vi "Pattern recognizer.vi"() -> ()   [LabVIEW 2020]
uses:
  <vilib>/Native 3D Graph/xcontrol/3DPC_SurfacePlot.xctl
  controls/Pattern recognizer data.ctl
  cc2a312d-b526-45fa-be19-77dd4eded1a7.vi
  <vilib>/measure/mamon.llb/Waveform Peak Detection for 1 Chan.vi
  <vilib>/measure/NI_MAPro.lvlib
panel:
  in  "Tab Control":enum32{"Load", "Analyse"}(tab)
  in  "Messages":string
  in  "Fast load":bool=TRUE
  in  "Stop":bool
  out "Slicer view":cluster{"X":dbl, "Y":dbl}[](graph)
  in  "File Path":path
  in  "Load":bool
  out "3D Graph":refnum<class "Base Datatype.lvclass">[](xcontrol)
  in  "Width":i32=2
  in  "peaks/valleys":enum16{"Peaks", "Valleys"}(ring)
  in  "Threshold":dbl
  in  "Previous":bool
  in  "Next":bool
  in  "Loop count (0 for continuous)":u32
  in  "Generate":bool
  in  "Layer #":cluster{"Numeric":u32, "Numeric":u32}(slide)={"Numeric"=0, "Numeric"=480} scale=0.0..480.0
  out "Line# end":u32
  out "Line# start":u32
  out "End Gcode":string
  in  "Pattern":T1(ring)
  out "Pattern view":cluster{dbl[], dbl[]}[](graph)
  out "Start Gcode":string
  in  "Close":bool
  # "EXPERIMENTAL! Works like sh*t"
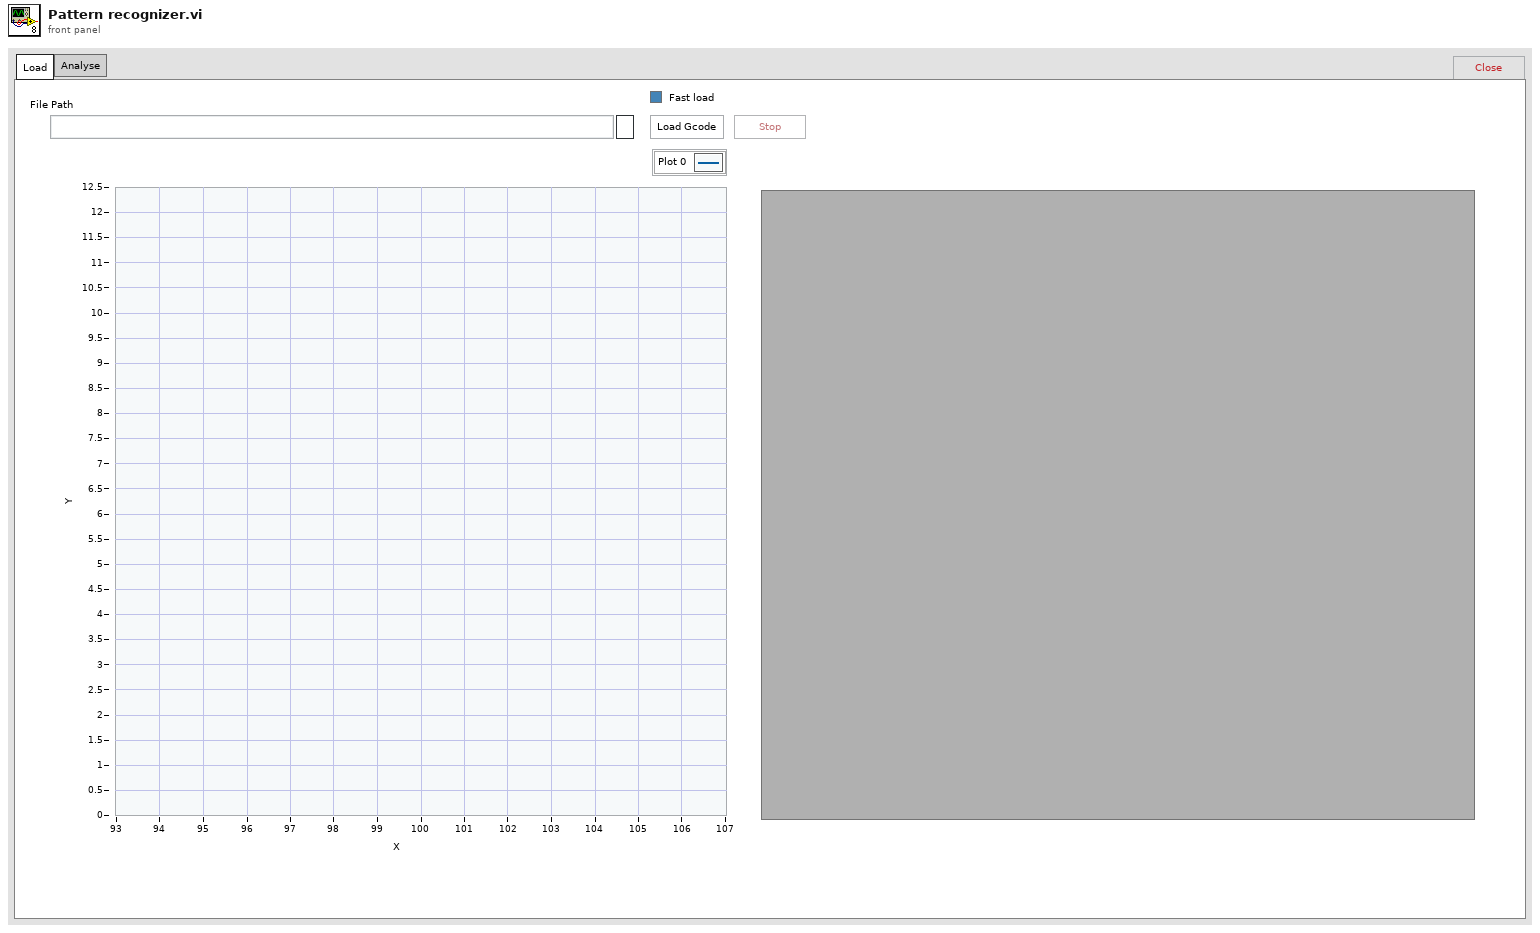
[diagram p1: front panel]
types:
  T1 = enum16{"X cumulative", "Y cumulative", "E cumulative", "X-Y absolute"}
  T2 = typedef "Pattern recognizer data.ctl" = cluster{"Gcode Array":string[], "Cumulative X":dbl[], "Cumulative Y":dbl[], "Cumulative E":dbl[], "Layer numbers":i32[], "Line number per layer":i32[]}
  T3 = enum8{"Enabled", "Disabled", "Disabled and Grayed Out"}
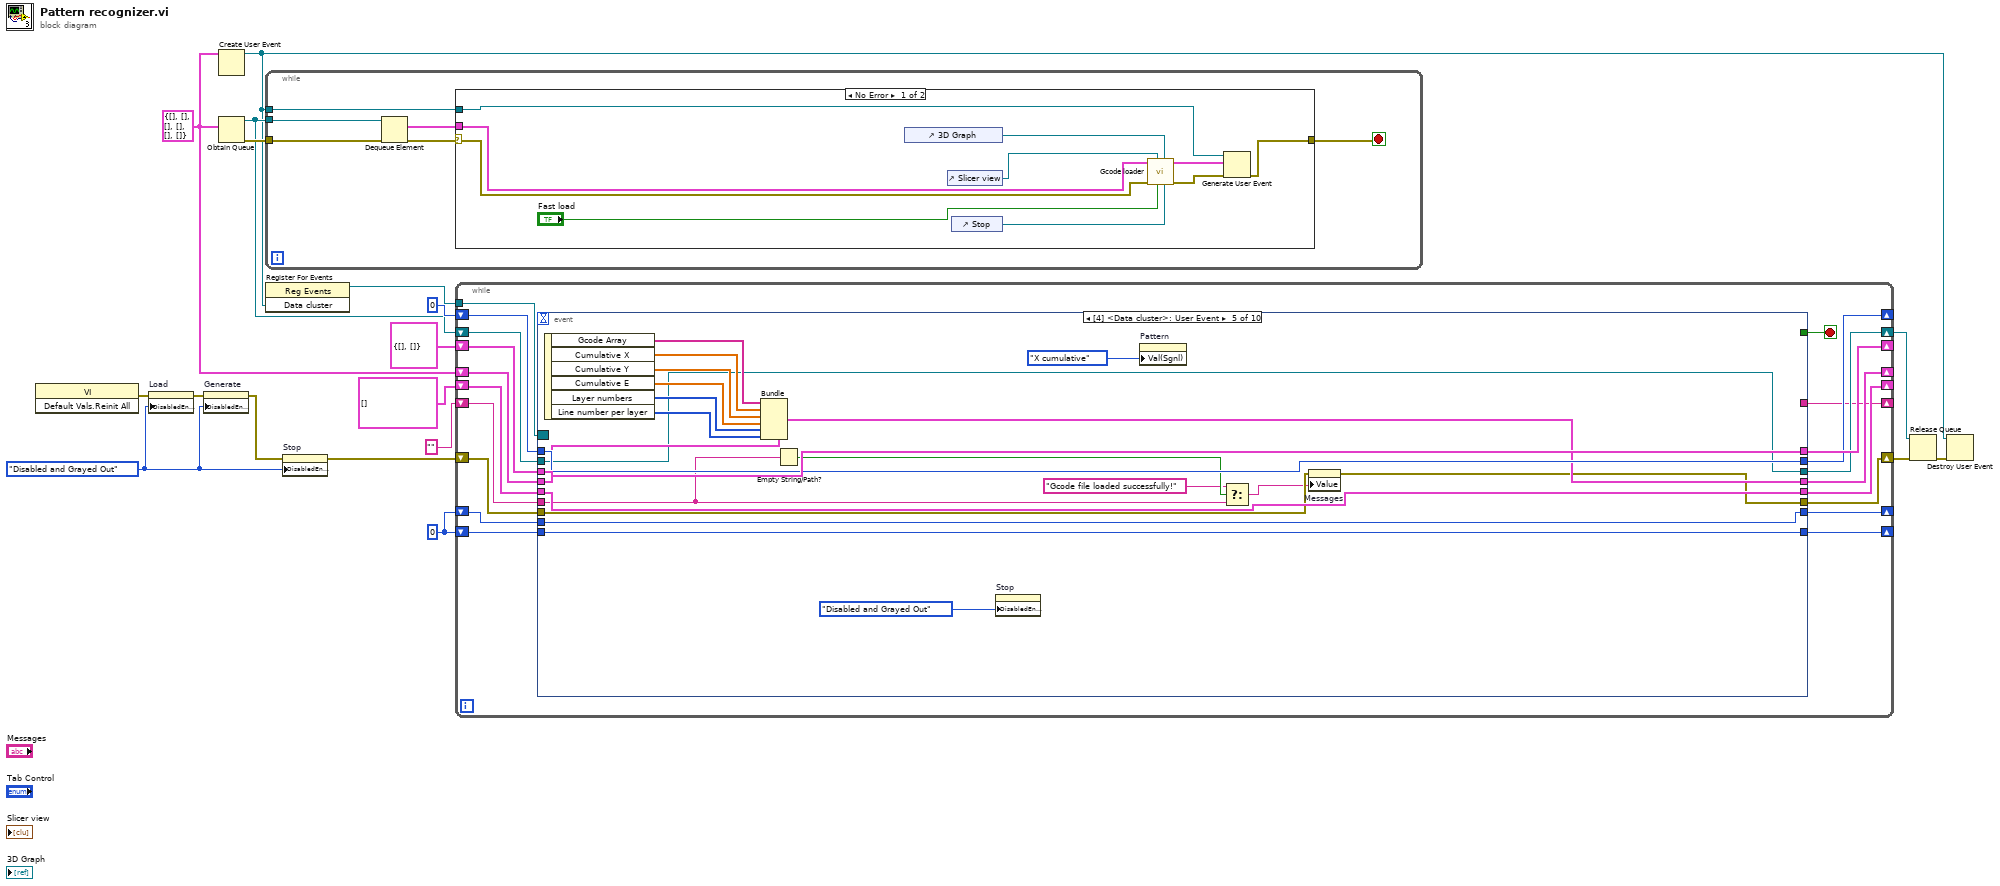
[diagram p0: block diagram]
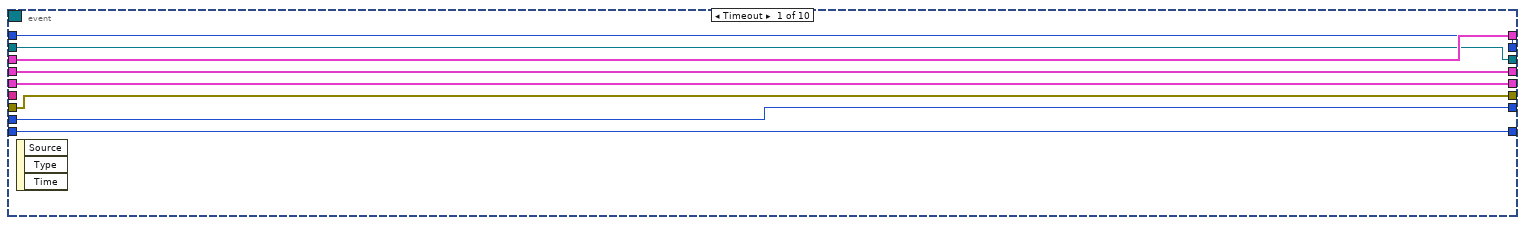
[diagram p3: hidden frame]
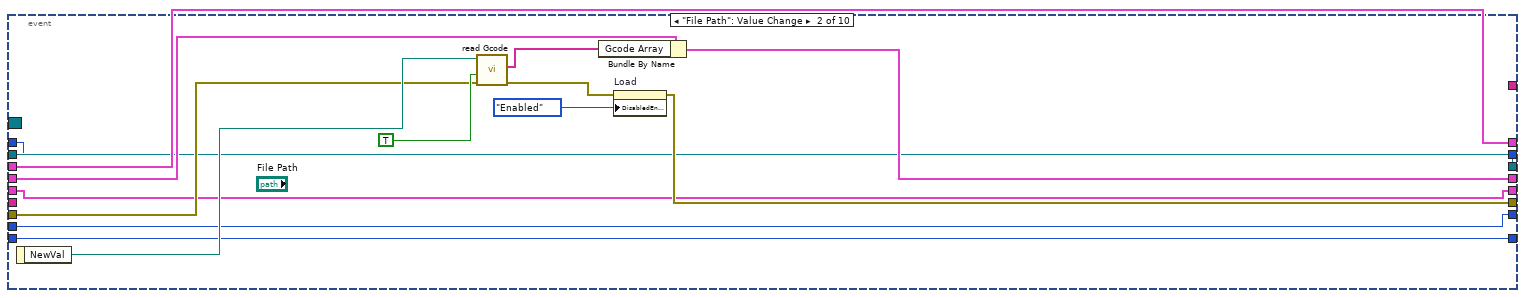
[diagram p4: hidden frame]
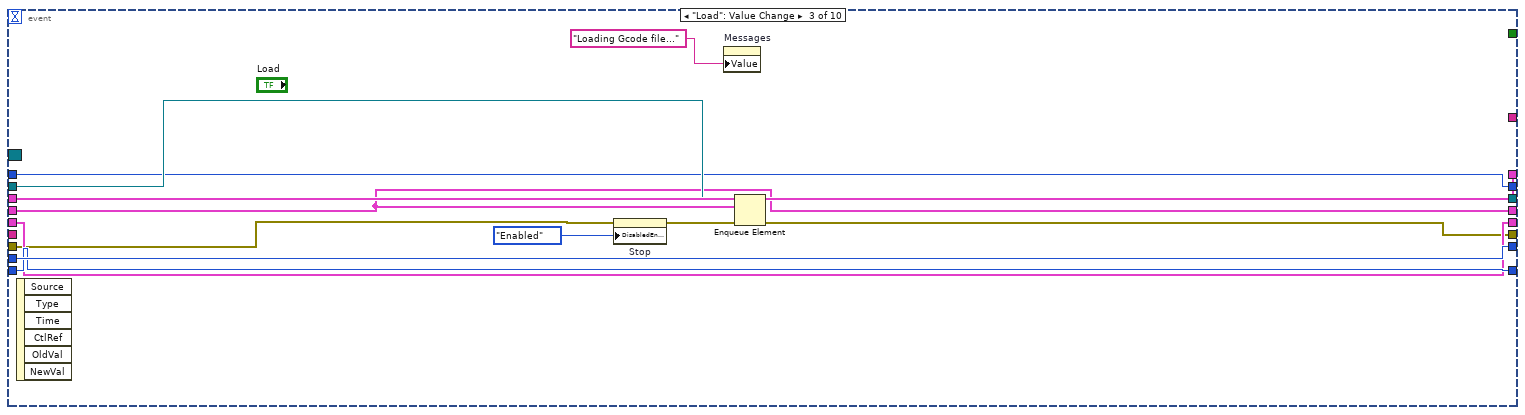
[diagram p5: hidden frame]
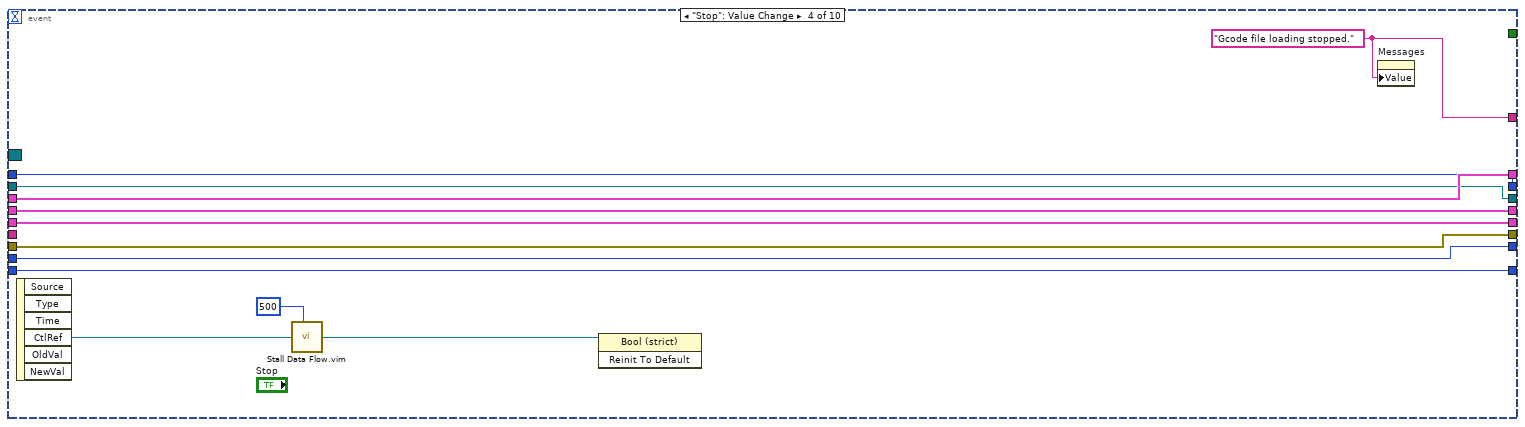
[diagram p6: hidden frame]
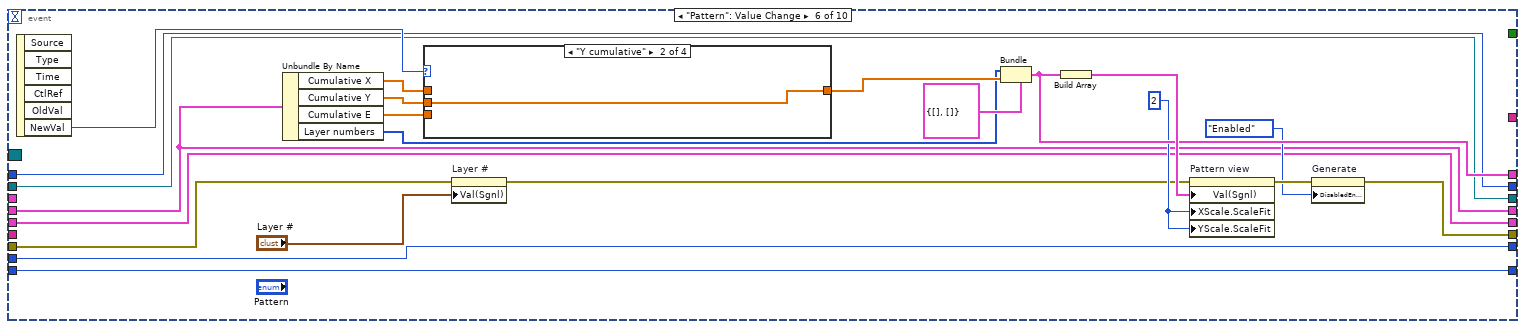
[diagram p7: hidden frame]
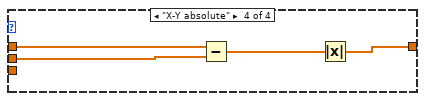
[diagram p10: hidden frame]
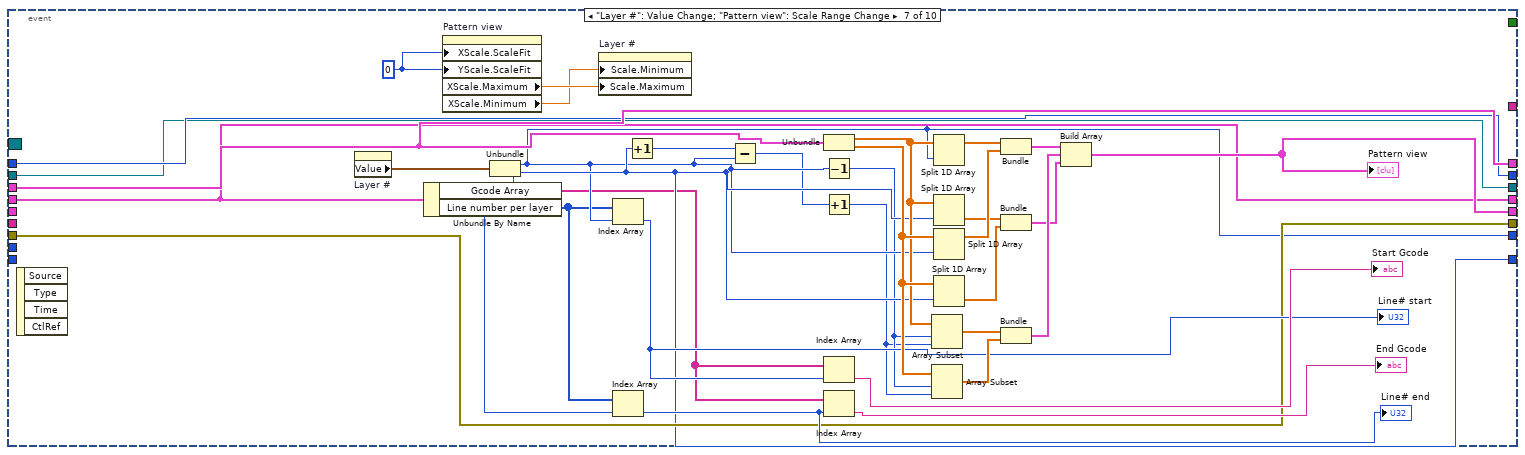
[diagram p11: hidden frame]
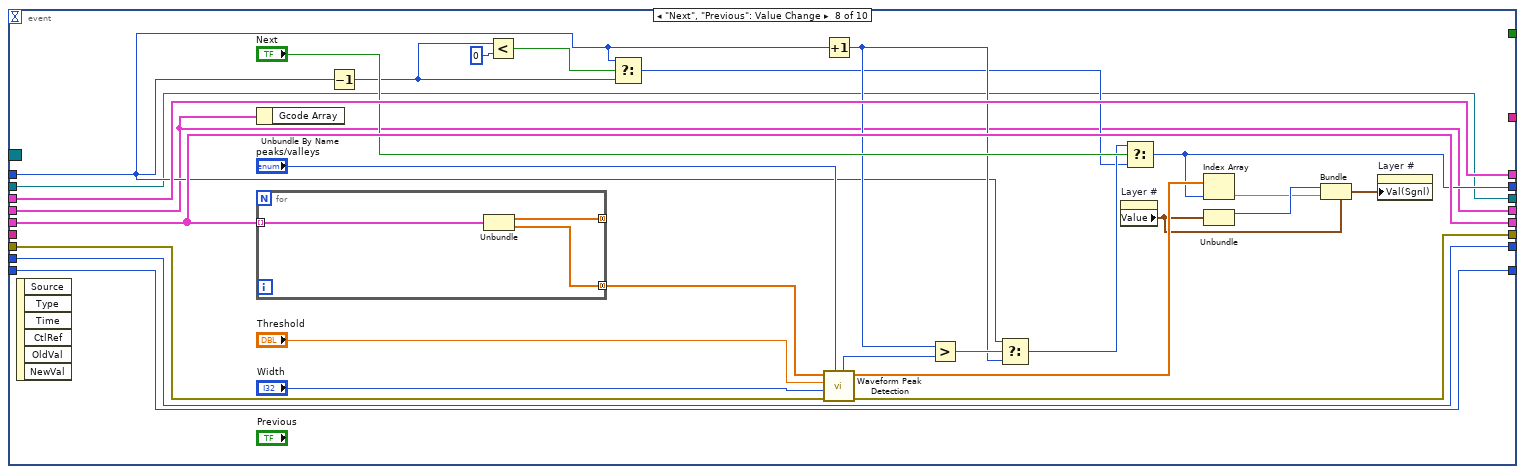
[diagram p12: hidden frame]
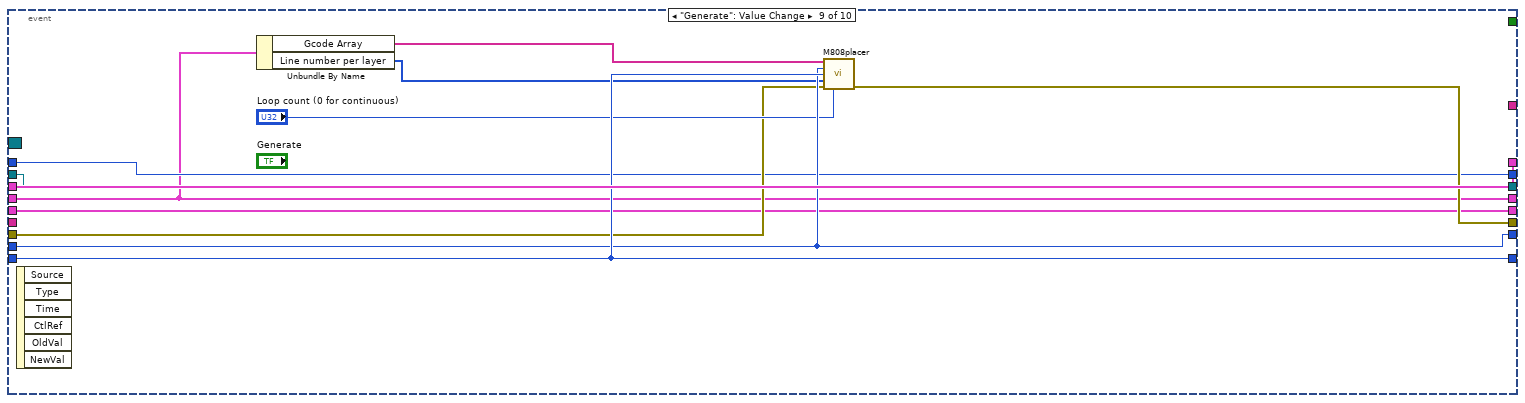
[diagram p13: hidden frame]
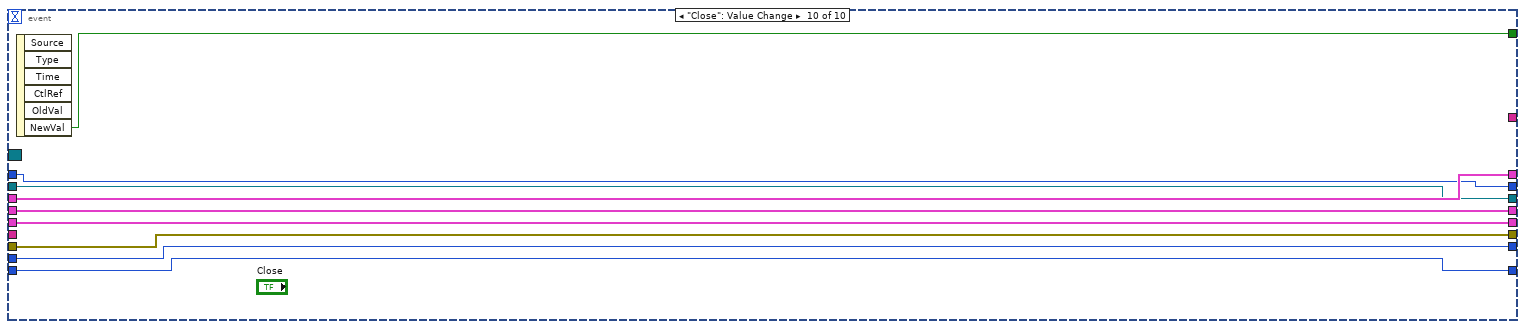
[diagram p14: hidden frame]
diagram:
  w11 = T2 {"Gcode Array"=[], "Cumulative X"=[], "Cumulative Y"=[], "Cumulative E"=[], "Layer numbers"=[], "Line number per layer"=[]} ("Data cluster")
  w3 = T3."Disabled and Grayed Out" ("Disabled")
  w17 = 0
  n1 = invoke class="VI" method="Default Vals.Reinit All"() -> (error out=w16:errorcluster)  [unwired: 3 in, 2 out]
  n2 = property on="Load" class="Bool"(error in=w16, "DisabledEnum"=w3) -> (error out=w15:errorcluster)  [unwired: 1 in, 1 out]
  n3 = property on="Generate" class="Bool"(error in=w15, "DisabledEnum"=w3) -> (error out=w2:errorcluster)  [unwired: 1 in, 1 out]
  n4 = Obtain Queue(element data type=w11) -> (queue out=w9:refnum<queue>, error out=w12:errorcluster)  [unwired: 4 in, 1 out]
  n5 = Create User Event(user event datatype=w11) -> (user event=w5:refnum<user-event>)  [unwired: 1 in, 1 out]
  n6 = while {
    tunnel: w9 -> [w24]
    tunnel: w12 -> [w23]
    tunnel: w5 -> [w19]
    stop <- w20 stop-if-true
    n7 = Dequeue Element(queue=w24, error in (no error)=w23) -> (element=w22:T2, error out=w21:errorcluster)  [unwired: 1 in, 2 out]
    n8 = case shown="No Error" w21 {
      selector: w21 -> [w33 w35]
      tunnel: w22 -> [w34 _]
      tunnel: [w27 w35] -> w20
      tunnel: w19 -> [w29 _]
      frame No Error {
        n9 = control-ref of="3D Graph"() -> (w32:refnum<vi>)
        n10 = control-ref of="Slicer view"() -> (w31:refnum<vi>)
        n11 = control-ref of="Stop"() -> (w26:refnum<vi>)
        n12 = call "Gcode loader.vi"("Stop"=w26, "3D Graph"=w32, "Fast load"="Fast load", "XYGraph in"=w31, "error in (no error)"=w33, "Data cluster"=w34) -> ("error out"=w30:errorcluster, "Data cluster out"=w28:T2)  [unwired: 4 in]
        n13 = Generate User Event(user event=w29, event data cluster=w28, error in=w30) -> (error out=w27:errorcluster)  [unwired: 1 in, 1 out]
      }
      frame Error {
      }
    }
  }
  n14 = register-events(w5) -> (reference out=w10:refnum<event-registration>)  [unwired: 2 in, 1 out]
  n15 = property on="Stop" class="Bool (strict)"(error in=w2, "DisabledEnum"=w3) -> (error out=w1:errorcluster)  [unwired: 1 in, 1 out]
  n16 = while {
    shift-right: [w54] -> _
    shift-left: cluster{dbl[], dbl[]} {[], []} -> [w53]
    shift-right: [w52] -> _
    shift-left: w17 -> [w50]
    shift-right: [w51] -> _
    shift-left: w17 -> [w49]
    shift-right: [w47] -> w7
    shift-left: w1 -> [w48]
    shift-right: [w46] -> _
    shift-left: cluster{dbl[], dbl[]}[] [] -> [w45]
    shift-right: [w43] -> _
    shift-left: 0 -> [w44]
    shift-right: [w41] -> _
    shift-left: w11 -> [w42]
    tunnel: w10 -> [w40]
    shift-right: [w38] -> w8
    shift-left: w9 -> [w39]
    shift-right: [w37] -> _
    shift-left: "" ("Messages") -> [w36]
    stop <- w55 stop-if-true
    n17 = event shown="[4] <Data cluster>: User Event" {
      selector: w40 -> [_ _ _ _ _ _ _ _ _ _]
      dyn-events: _ -> [_ _ _ _ _ _ _ _ _ _]
      timeout: _ -> [_ _ _ _ _ _ _ _ _ _]
      tunnel: [_ _ _ _ _ _ _ _ _ w239] -> w55
      tunnel: [w63 w77 w91 w103 w125 w143 w178 w215 w230 w238] -> w54
      tunnel: w53 -> [w63 w77 w91 w103 w125 _ w178 w215 w230 w238]
      tunnel: [w62 w75 w90 w102 w124 w139 w163 w214 w228 w237] -> w52
      tunnel: [w61 w74 w89 w101 w123 w138 w164 w213 w229 w236] -> w51
      tunnel: w50 -> [w62 w75 w90 w102 w124 w139 _ w214 w228 w237]
      tunnel: w49 -> [w61 w74 w89 w101 w123 w138 _ w213 w229 w236]
      tunnel: w48 -> [w60 w73 w80 w100 w110 w135 w167 w209 w226 w235]
      tunnel: [w60 w70 w85 w100 w109 w134 w167 w208 w225 w235] -> w47
      tunnel: [w59 w69 w88 w99 w122 w133 w166 w210 w224 w234] -> w46
      tunnel: w45 -> [w59 w69 w88 w99 w122 w133 _ w210 w224 w234]
      tunnel: w44 -> [w58 w64 w83 w98 w121 w132 w165 w202 w223 w233]
      tunnel: [w58 w64 w83 w98 w121 w132 w165 w192 w223 w233] -> w43
      tunnel: w42 -> [w57 w68 w86 w97 w120 w131 w157 w189 w222 w232]
      tunnel: [w57 w66 w86 w97 w113 w131 w157 w189 w222 w232] -> w41
      tunnel: w39 -> [w56 w65 w87 w96 w111 w126 w155 w188 w219 w231]
      tunnel: [w56 w65 w84 w96 w111 w126 w155 w188 w219 w231] -> w38
      tunnel: [_ _ _ w92 _ _ _ _ _ _] -> w37
      tunnel: w36 -> [_ _ _ _ w105 _ _ _ _ _]
      event Timeout {
        n18 = event-data() -> ()  [unwired: 1 in, 3 out]
      }
      event "File Path": Value Change {
        n19 = event-data() -> ("NewVal"=w78:path)  [unwired: 1 in]
        n20 = call "read Gcode.vi"("error in"=w73, "Parse comment lines"=TRUE, "Gcode path (use dialog)"=w78) -> ("error out"=w71:errorcluster, "Gcode Array"=w67:string[])  [unwired: 6 in, 1 out]
        n21 = Bundle By Name(cluster=w68, "Gcode Array"=w67) -> (w66:T2)
        n22 = property on="Load" class="Bool"(error in=w71, "DisabledEnum"=T3."Enabled" ("Disabled")) -> (error out=w70:errorcluster)  [unwired: 1 in, 1 out]
      }
      event "Load": Value Change {
        n23 = event-data() -> ()  [unwired: 1 in, 6 out]
        n24 = property on="Stop" class="Bool (strict)"(error in=w80, "DisabledEnum"=T3."Enabled" ("Disabled")) -> (error out=w79:errorcluster)  [unwired: 1 in, 1 out]
        n25 = property on="Messages" class="Str"("Value"="Loading Gcode file..." ("Messages")) -> ()  [unwired: 2 in, 2 out]
        n26 = Enqueue Element(queue=w87, element=w86, error in (no error)=w79) -> (queue out=w84:refnum<queue>, error out=w85:errorcluster)  [unwired: 1 in, 1 out]
      }
      event "Stop": Value Change {
        w92 = "Gcode file loading stopped." ("Messages")
        n27 = event-data() -> ("CtlRef"=w95:refnum<vi>)  [unwired: 1 in, 5 out]
        n28 = call "Stall Data Flow.vim"("value in"=w95, "milliseconds to wait"=u32 500) -> ("value out"=w94:refnum<vi>)  [unwired: 1 out]
        n29 = invoke class="Bool (strict)" method="Reinit To Default"(reference=w94) -> ()  [unwired: 2 in, 3 out]
        n30 = property on="Messages" class="Str"("Value"=w92) -> ()  [unwired: 2 in, 2 out]
      }
      event User Event {
        n31 = event-data() -> ("Gcode Array"=w119:string[], "Cumulative X"=w118:dbl[], "Cumulative Y"=w117:dbl[], "Cumulative E"=w116:dbl[], "Layer numbers"=w115:i32[], "Line number per layer"=w114:i32[])  [unwired: 1 in]
        n32 = Bundle(cluster=w120, "Gcode Array"=w119, "Cumulative X"=w118, "Cumulative Y"=w117, "Cumulative E"=w116, "Layer numbers"=w115, "Line number per layer"=w114) -> (w113:T2)
        n33 = Empty String/Path?(string/path=w105) -> (empty?=w108:bool)
        n34 = property on="Stop" class="Bool (strict)"("DisabledEnum"=T3."Disabled and Grayed Out" ("Disabled")) -> ()  [unwired: 2 in, 2 out]
        n35 = property on="Pattern" class="Enum (strict)"("Val(Sgnl)"=T1."X cumulative" ("Value (Signaling)")) -> ()  [unwired: 2 in, 2 out]
        n36 = Select(t="Gcode file loaded successfully!" ("Messages"), s=w108, f=w105) -> (s? t:f=w106:string)
        n37 = property on="Messages" class="Str"(error in=w110, "Value"=w106) -> (error out=w109:errorcluster)  [unwired: 1 in, 1 out]
      }
      event "Pattern": Value Change {
        w142 = u8 2 ("X Scale.Scale Fit")
        n38 = event-data() -> ("NewVal"=w147:T1)  [unwired: 1 in, 5 out]
        n39 = Unbundle By Name(w131) -> ("Cumulative X"=w130:dbl[], "Cumulative Y"=w129:dbl[], "Cumulative E"=w128:dbl[], "Layer numbers"=w127:i32[])
        n40 = case shown="\"Y cumulative\"" w147 {
          tunnel: [w148 w149 w150 w151] -> w145
          tunnel: w130 -> [w148 _ _ w154]
          tunnel: w129 -> [_ w149 _ w153]
          tunnel: w128 -> [_ _ w150 _]
          frame "X cumulative", Default {
          }
          frame "Y cumulative" {
          }
          frame "E cumulative" {
          }
          frame "X-Y absolute" {
            n41 = Subtract(x=w154, y=w153) -> (x-y=w152:dbl[])
            n42 = Absolute Value(x=w152) -> (abs(x)=w151:dbl[])
          }
        }
        n43 = property on="Layer #" class="Slide (strict)"(error in=w135, "Val(Sgnl)"="Layer #") -> (error out=w140:errorcluster)  [unwired: 1 in, 1 out]
        n44 = Bundle(cluster=cluster{dbl[], dbl[]} {[], []}, w127, w145) -> (w143:cluster{dbl[], dbl[]})
        n45 = Build Array(w143) -> (w144:cluster{dbl[], dbl[]}[])
        n46 = property on="Pattern view" class="XYGraph (strict)"(error in=w140, "Val(Sgnl)"=w144, "XScale.ScaleFit"=w142, "YScale.ScaleFit"=w142) -> (error out=w137:errorcluster)  [unwired: 1 in, 1 out]
        n47 = property on="Generate" class="Bool"(error in=w137, "DisabledEnum"=T3."Enabled" ("Disabled")) -> (error out=w134:errorcluster)  [unwired: 1 in, 1 out]
      }
      event "Layer #": Value Change; "Pattern view": Scale Range Change {
        w175 = u8 0 ("X Scale.Scale Fit")
        n48 = event-data() -> ()  [unwired: 1 in, 4 out]
        n49 = property on="Layer #" class="Slide (strict)"() -> ("Value"=w172:cluster{"Numeric":u32, "Numeric":u32})  [unwired: 2 in, 2 out]
        n50 = Unbundle By Name(w157) -> ("Gcode Array"=w158:string[], "Line number per layer"=w156:i32[])
        n51 = property on="Pattern view" class="XYGraph (strict)"("XScale.ScaleFit"=w175, "YScale.ScaleFit"=w175) -> ("XScale.Maximum"=w174:dbl, "XScale.Minimum"=w173:dbl)  [unwired: 2 in, 2 out]
        n52 = Unbundle(w172) -> ("Numeric"=w163:u32, "Numeric"=w164:u32)
        n53 = property on="Layer #" class="Slide (strict)"("Scale.Minimum"=w173, "Scale.Maximum"=w174) -> ()  [unwired: 2 in, 2 out]
        n54 = Index Array(array=w156, index=w163) -> (element=w169:i32)
        "Line# start" <- w169
        n55 = Index Array(array=w156, index=w164) -> (element=w168:i32)
        "Line# end" <- w168
        n56 = Increment(x=w164) -> (x+1=w161:u32)
        n57 = Subtract(x=w161, y=w163) -> (x-y=w162:u32)
        n58 = Unbundle(w178) -> (w176:dbl[], w177:dbl[])
        n59 = Decrement(x=w163) -> (x-1=w160:u32)
        n60 = Increment(x=w162) -> (x+1=w159:u32)
        n61 = Index Array(array=w158, index=w169) -> (element=→"Start Gcode":string)
        n62 = Index Array(array=w158, index=w168) -> (element=→"End Gcode":string)
        n63 = Array Subset(array=w176, index=w160, length=w159) -> (w180:dbl[])
        n64 = Array Subset(array=w177, index=w160, length=w159) -> (w179:dbl[])
        n65 = Split 1D Array(array=w176, index=w163) -> (first subarray=w187:dbl[])  [unwired: 1 out]
        n66 = Split 1D Array(array=w176, index=w164) -> (second subarray=w185:dbl[])  [unwired: 1 out]
        n67 = Split 1D Array(array=w177, index=w163) -> (first subarray=w186:dbl[])  [unwired: 1 out]
        n68 = Split 1D Array(array=w177, index=w164) -> (second subarray=w184:dbl[])  [unwired: 1 out]
        n69 = Bundle(w187, w186) -> (w183:cluster{dbl[], dbl[]})  [unwired: 1 in]
        n70 = Bundle(w185, w184) -> (w181:cluster{dbl[], dbl[]})  [unwired: 1 in]
        n71 = Bundle(w180, w179) -> (w182:cluster{dbl[], dbl[]})  [unwired: 1 in]
        n72 = Build Array(w183, w182, w181) -> (w166:cluster{dbl[], dbl[]}[])
        "Pattern view" <- w166
      }
      event "Next", "Previous": Value Change {
        n73 = event-data() -> ()  [unwired: 1 in, 6 out]
        n74 = Unbundle By Name(w189) -> ()  [unwired: 1 out]
        n75 = for {
          tunnel: w210 -> [w218] mode=indexing
          tunnel: [w217] -> w194 mode=concatenating
          tunnel: [w216] -> _ mode=concatenating
          n76 = Unbundle(w218) -> (w216:dbl[], w217:dbl[])
        }
        n77 = Decrement(x=w202) -> (x-1=w203:i32)
        n78 = Less?(x=w203, y=0) -> (x < y?=w205:bool)
        n79 = Select(t=w202, s=w205, f=w203) -> (s? t:f=w200:i32)
        n80 = Increment(x=w202) -> (x+1=w204:i32)
        n81 = call-poly <vilib>:"Waveform Peak Detection.vi"("peaks/valleys"="peaks/valleys", "error in"=w209, "width"="Width", "threshold"="Threshold", "Signal In"=w194) -> ("error out"=w208:errorcluster, "Locations"=w199:dbl[], "# found"=w193:i32)  [unwired: 2 in, 2 out]
        n82 = Greater?(x=w204, y=w193) -> (0:w206:bool)
        n83 = Select(t=w202, s=w206, f=w204) -> (s? t:f=w201:i32)
        n84 = property on="Layer #" class="Slide (strict)"() -> ("Value"=w197:cluster{"Numeric":u32, "Numeric":u32})  [unwired: 2 in, 2 out]
        n85 = Select(t=w201, s="Next", f=w200) -> (s? t:f=w192:i32)
        n86 = Index Array(array=w199, index=w192) -> (element=w191:dbl)
        n87 = Unbundle(w197) -> ("Numeric"=w198:u32)  [unwired: 1 out]
        n88 = Bundle(cluster=w197, "Numeric"=w198, "Numeric"=w191) -> (w196:cluster{"Numeric":u32, "Numeric":u32})
        n89 = property on="Layer #" class="Slide (strict)"("Val(Sgnl)"=w196) -> ()  [unwired: 2 in, 2 out]
      }
      event "Generate": Value Change {
        n90 = event-data() -> ()  [unwired: 1 in, 6 out]
        n91 = Unbundle By Name(w222) -> ("Gcode Array"=w221:string[], "Line number per layer"=w220:i32[])
        n92 = call "M808placer.vi"("Gcode Array in"=w221, "Line # start"=w228, "Line # end"=w229, "Gcode line # array in"=w220, "error in"=w226, "Loop count"="Loop count (0 for continuous)") -> ("error out"=w225:errorcluster)  [unwired: 8 in, 1 out]
      }
      event "Close": Value Change {
        n93 = event-data() -> ("NewVal"=w239:bool)  [unwired: 1 in, 5 out]
      }
    }
  }
  n94 = Release Queue(queue=w8, error in (no error)=w7) -> (error out=w6:errorcluster)  [unwired: 1 in, 2 out]
  n95 = Destroy User Event(user event=w5, error in=w6) -> ()  [unwired: 1 out]
